vi "CleanUp Diagram.vi"(8 "error in (no error)":errorcluster, 10 "Top Level Diagram":refnum<vi>, 11 "Loop in":refnum<class "Loop.lvclass">) -> (0 "error out":errorcluster, 3 "Loop out":refnum<class "Loop.lvclass">)   [LabVIEW 2015, in "Loop.lvclass"]
uses:
  Loop.lvclass
  Structures/Structures.lvclass/Structures.ctl
  Loop.lvclass/Loop.ctl
  Structures/Read Structure.vi
  Read Loop Structure.vi
  Structures/Read Diagram.vi
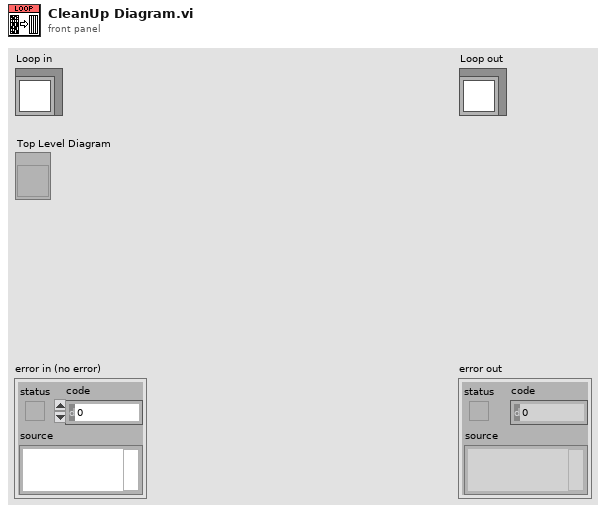
[diagram p1: front panel]
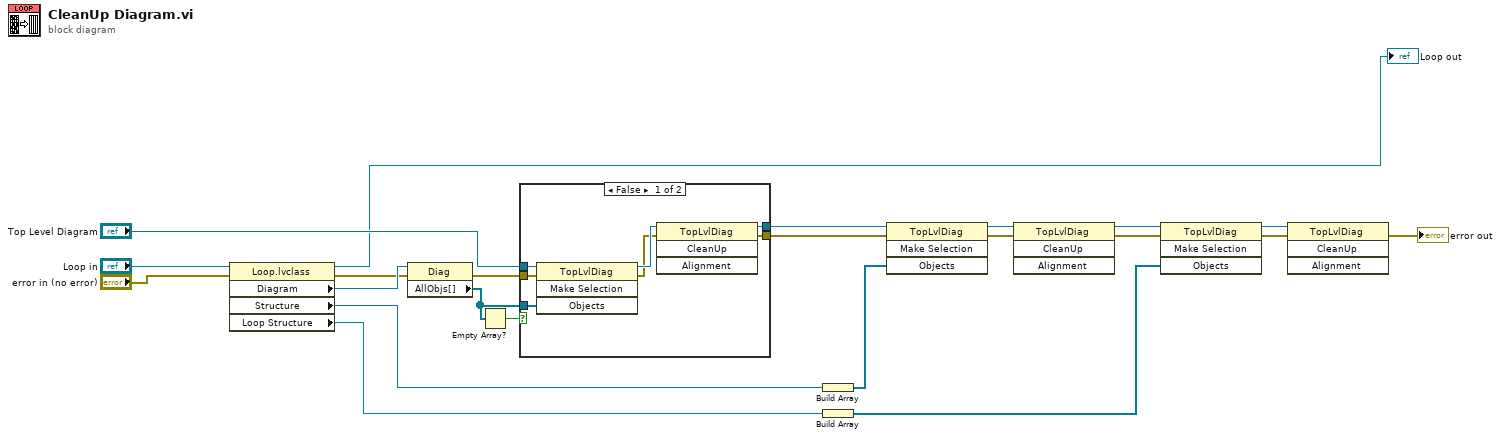
[diagram p0: block diagram]
diagram:
  n1 = property class="Loop.lvclass"(reference="Loop in", error in="error in (no error)") -> (reference out=→"Loop out":refnum<class "Loop.lvclass">, error out=w6:errorcluster, "Diagram"=w22:refnum<vi>, "Structure"=w7:refnum<vi>, "Loop Structure"=w9:refnum<vi>)
  n2 = property class="Diag"(reference=w22, error in=w6) -> (error out=w21:errorcluster, "AllObjs[]"=w17:refnum<vi>[])  [unwired: 1 out]
  n3 = Empty Array?(array=w17) -> (empty?=w16:bool)
  n4 = case shown="False" w16 {
    tunnel: "Top Level Diagram" -> [w29 w30]
    tunnel: w21 -> [w26 w31]
    tunnel: [w25 w31] -> w8
    tunnel: [w24 w30] -> w19
    tunnel: w17 -> [w23 _]
    frame False {
      n5 = invoke class="TopLvlDiag" method="Make Selection"(reference=w29, error in=w26, "Objects"=w23) -> (reference out=w28:refnum<vi>, error out=w27:errorcluster)  [unwired: 1 in, 2 out]
      n6 = invoke class="TopLvlDiag" method="CleanUp"(reference=w28, error in=w27) -> (reference out=w24:refnum<vi>, error out=w25:errorcluster)  [unwired: 2 in, 2 out]
    }
    frame True {
    }
  }
  n7 = Build Array(w7) -> (w15:refnum<vi>[])
  n8 = Build Array(w9) -> (w10:refnum<vi>[])
  n9 = invoke class="TopLvlDiag" method="Make Selection"(reference=w19, error in=w8, "Objects"=w15) -> (reference out=w18:refnum<vi>, error out=w20:errorcluster)  [unwired: 1 in, 2 out]
  n10 = invoke class="TopLvlDiag" method="CleanUp"(reference=w18, error in=w20) -> (reference out=w11:refnum<vi>, error out=w12:errorcluster)  [unwired: 2 in, 2 out]
  n11 = invoke class="TopLvlDiag" method="Make Selection"(reference=w11, error in=w12, "Objects"=w10) -> (reference out=w14:refnum<vi>, error out=w13:errorcluster)  [unwired: 1 in, 2 out]
  n12 = invoke class="TopLvlDiag" method="CleanUp"(reference=w14, error in=w13) -> (error out=→"error out":errorcluster)  [unwired: 2 in, 3 out]
